vi "Read Output Enable.vi"(11 "Signal Generator in":refnum<class "Vector Signal Generator.lvclass">) -> (2 "Output Enable":bool, 3 "Signal Generator out":refnum<class "Vector Signal Generator.lvclass">)   [LabVIEW 2020, in "Vector Signal Generator.lvclass"]
uses:
  Vector Signal Generator.lvclass
  Vector Signal Generator.lvclass/Vector Signal Generator.ctl
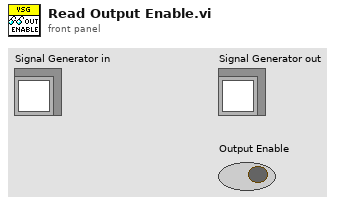
[diagram p1: front panel]
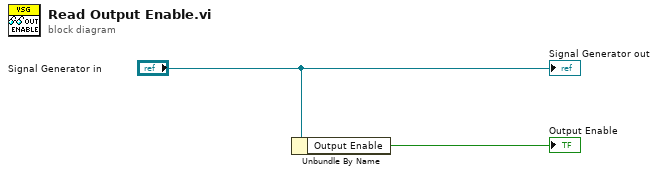
[diagram p0: block diagram]
diagram:
  n1 = Unbundle By Name("Signal Generator in") -> ("Output Enable"=→"Output Enable":bool)
  "Signal Generator out" <- "Signal Generator in"
